vi "修改-探头报警值-网络版.vi"(7 "模式":enum16{"单项", "批量"}(ring), 8 "error in (no error)":errorcluster caption="错误输入（无错误）", 11 "探头属性 i":T1) -> (0 "error out":errorcluster caption="错误输出", 1 "取消?":bool=TRUE, 3 "探头属性 o":T1)   [LabVIEW 2017]
panel:
  in  "静音延迟":u16=5 min=5
  in  "报警方式选择":enum16{"常报警", "自动静音", "手动静音"}(ring)
  in  "累积限值":dbl=0.5 min=0.0 max=65536.0 format="%#_6f"
  in  "硬件报警等级":enum16{"一级限值", "二级限值"}(ring)
  in  "限值2":sgl=0.5 min=0 max=6553.6 format="%#.2f"
  in  "单位2":enum8{"uSv/h", "mSv/h"}(ring)
  in  "取消按钮":bool
  in  "确定按钮":bool
  in  "限值1":sgl=0.5 min=0 max=6553.6 format="%#.2f"
  in  "单位1":enum8{"uSv/h", "mSv/h"}(ring)
  # "剂量率限值"
  # "一级报警限值"
  # "二级报警限值"
  # "探头报警限值"
  # "报警与静音"
  # "静音延迟(秒)"
  # "自然累积剂量限值"
  # "累积报警限值"
  # "mSv"
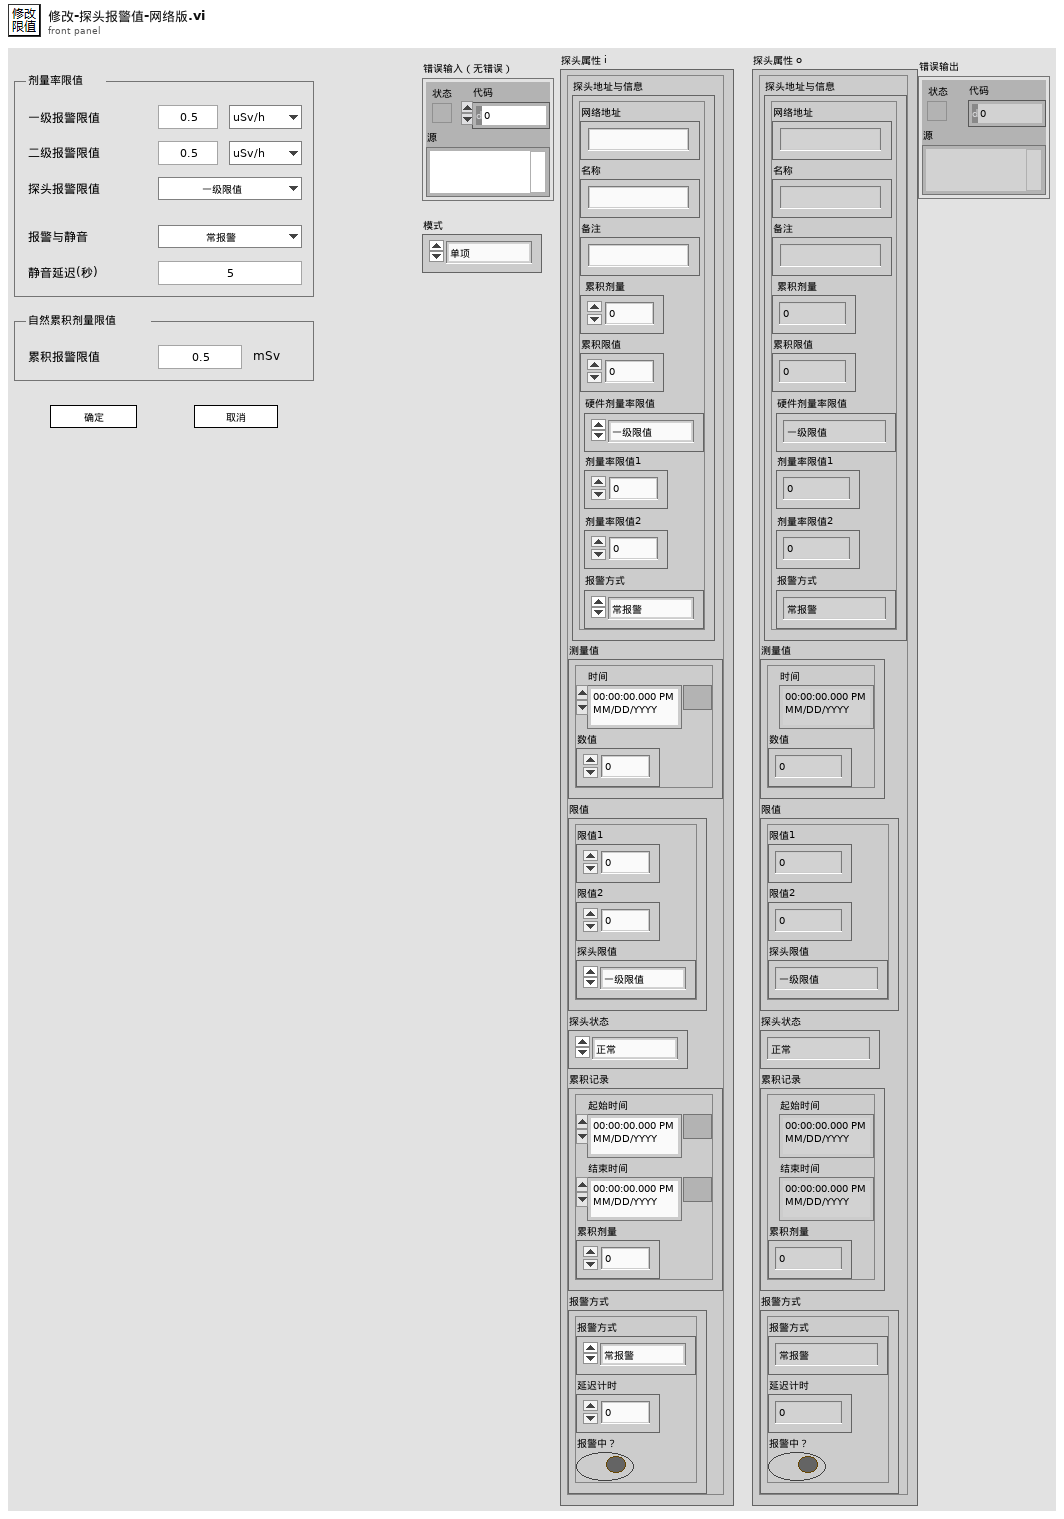
[diagram p1: front panel]
types:
  T1 = typedef "探头属性.ctl" = cluster{"探头地址与信息":T2, "测量值":T5, "限值":T6, "探头状态":T7, "累积记录":T8, "报警方式":T9}
  T2 = typedef "探测器信息.ctl" = cluster{"网络地址":string, "名称":string, "备注":string, "累积剂量":dbl, "累积限值":dbl, "硬件剂量率限值":T3, "剂量率限值1":dbl, "剂量率限值2":dbl, "报警方式":T4}
  T3 = typedef "探头剂量率限值选择.ctl" = enum16{"一级限值", "二级限值"}
  T4 = typedef "报警方式选择.ctl" = enum16{"常报警", "自动静音", "手动静音"}
  T5 = typedef "测量值.ctl" = cluster{"时间":timestamp, "数值":dbl}
  T6 = typedef "剂量率限值.ctl" = cluster{"限值1":dbl, "限值2":dbl, "探头限值":T3}
  T7 = typedef "探头状态.ctl" = enum16{"正常", "离线", "禁用", "一级报警", "二级报警", "累积报警"}
  T8 = typedef "单条累积记录.ctl" = cluster{"起始时间":timestamp, "结束时间":timestamp, "累积剂量":dbl}
  T9 = typedef "报警方式.ctl" = cluster{"报警方式":T4, "延迟计时":u16, "报警中？":bool}
  T10 = enum32{"Invalid", "Standard", "Closed", "Hidden", "Minimized", "Maximized"}
  T11 = enum8{"Enabled", "Disabled", "Disabled and Grayed Out"}
  T12 = typedef "簇-输入.ctl" = cluster{"配置文件动作":T13, "数据输入":variant}
  T13 = typedef "枚举-配置文件动作.ctl" = enum16{"初始化加载配置", "读取配置", "写入-屏幕键盘", "写入-静音延迟", "写入-主要探头类型", "写入-串口配置", "写入-累积定时", "写入-导出定时", "保存配置到文件"}
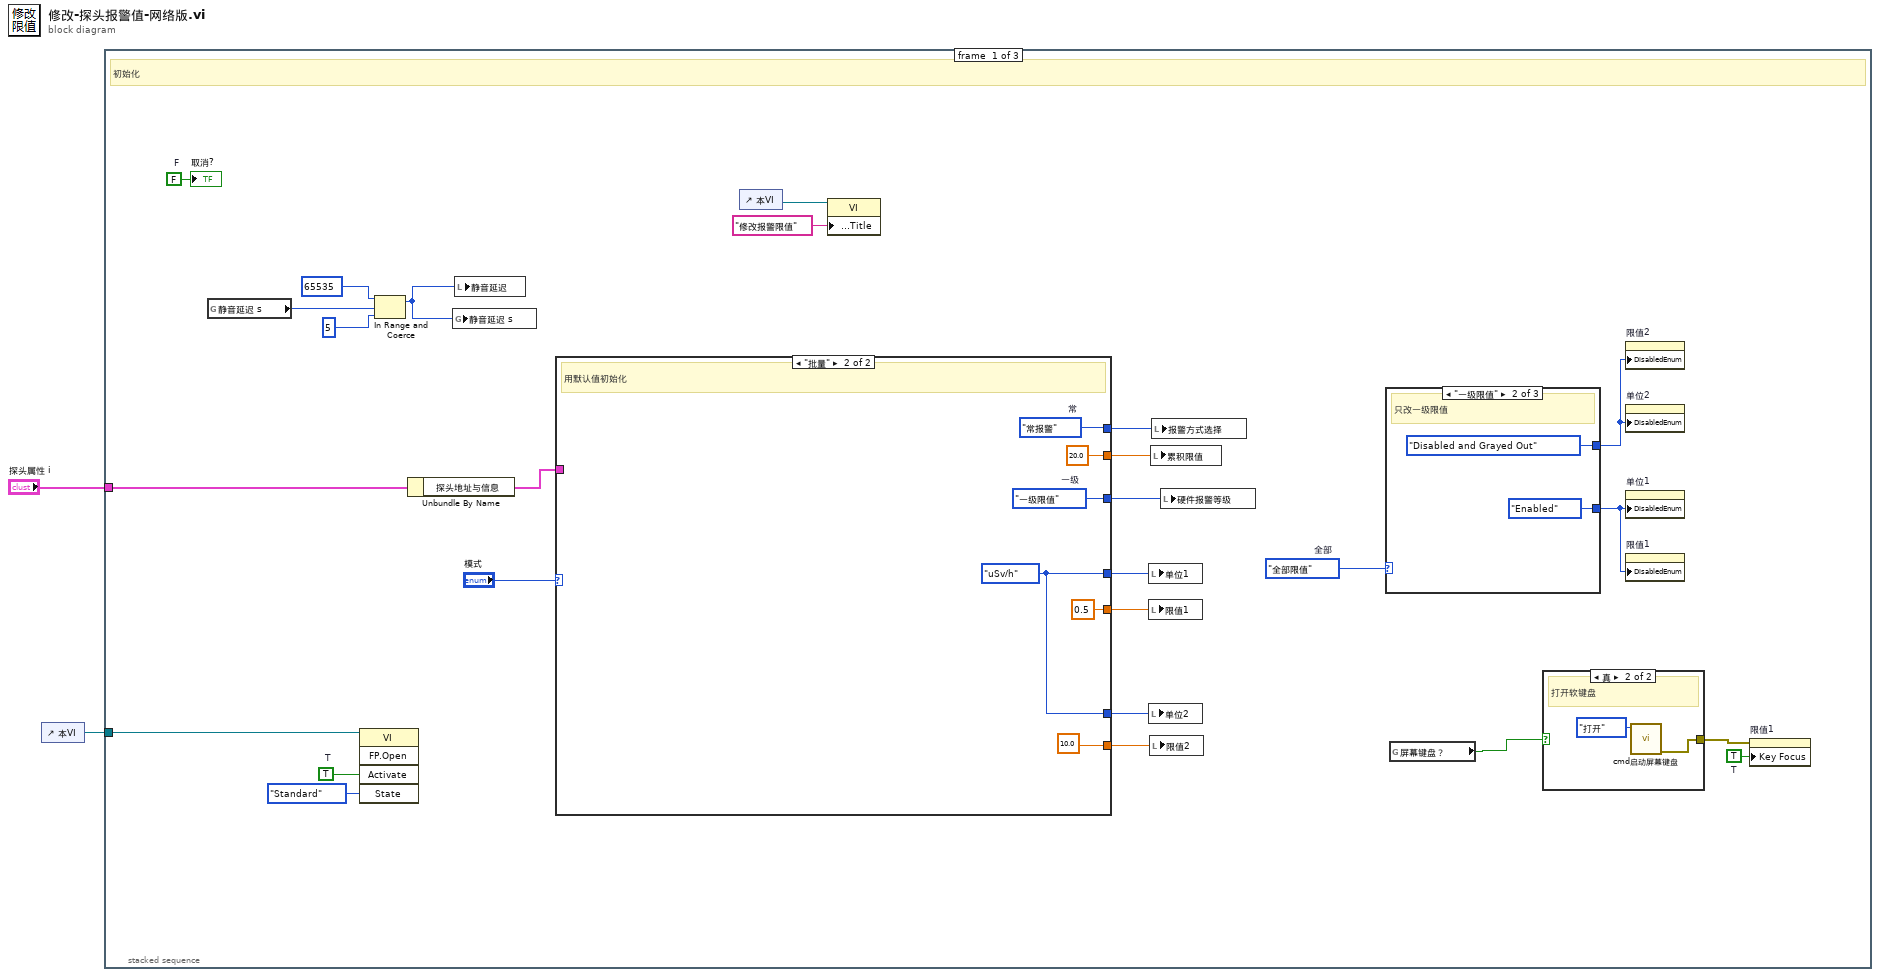
[diagram p0: block diagram]
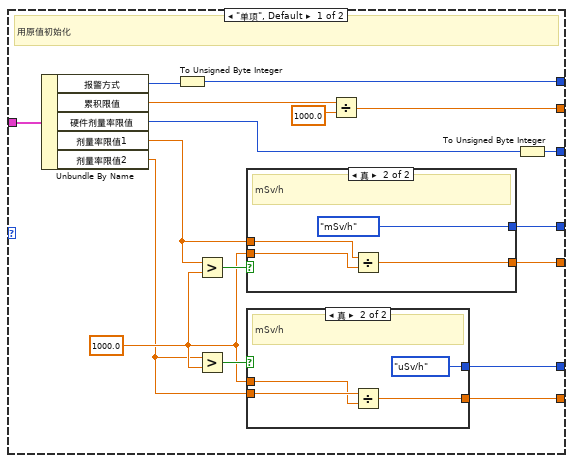
[diagram p2: hidden frame]
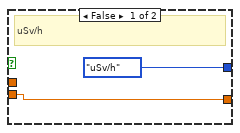
[diagram p3: hidden frame]
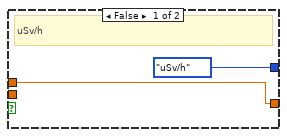
[diagram p4: hidden frame]
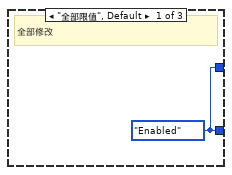
[diagram p6: hidden frame]
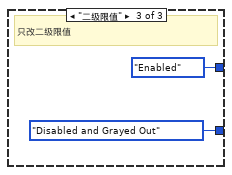
[diagram p7: hidden frame]
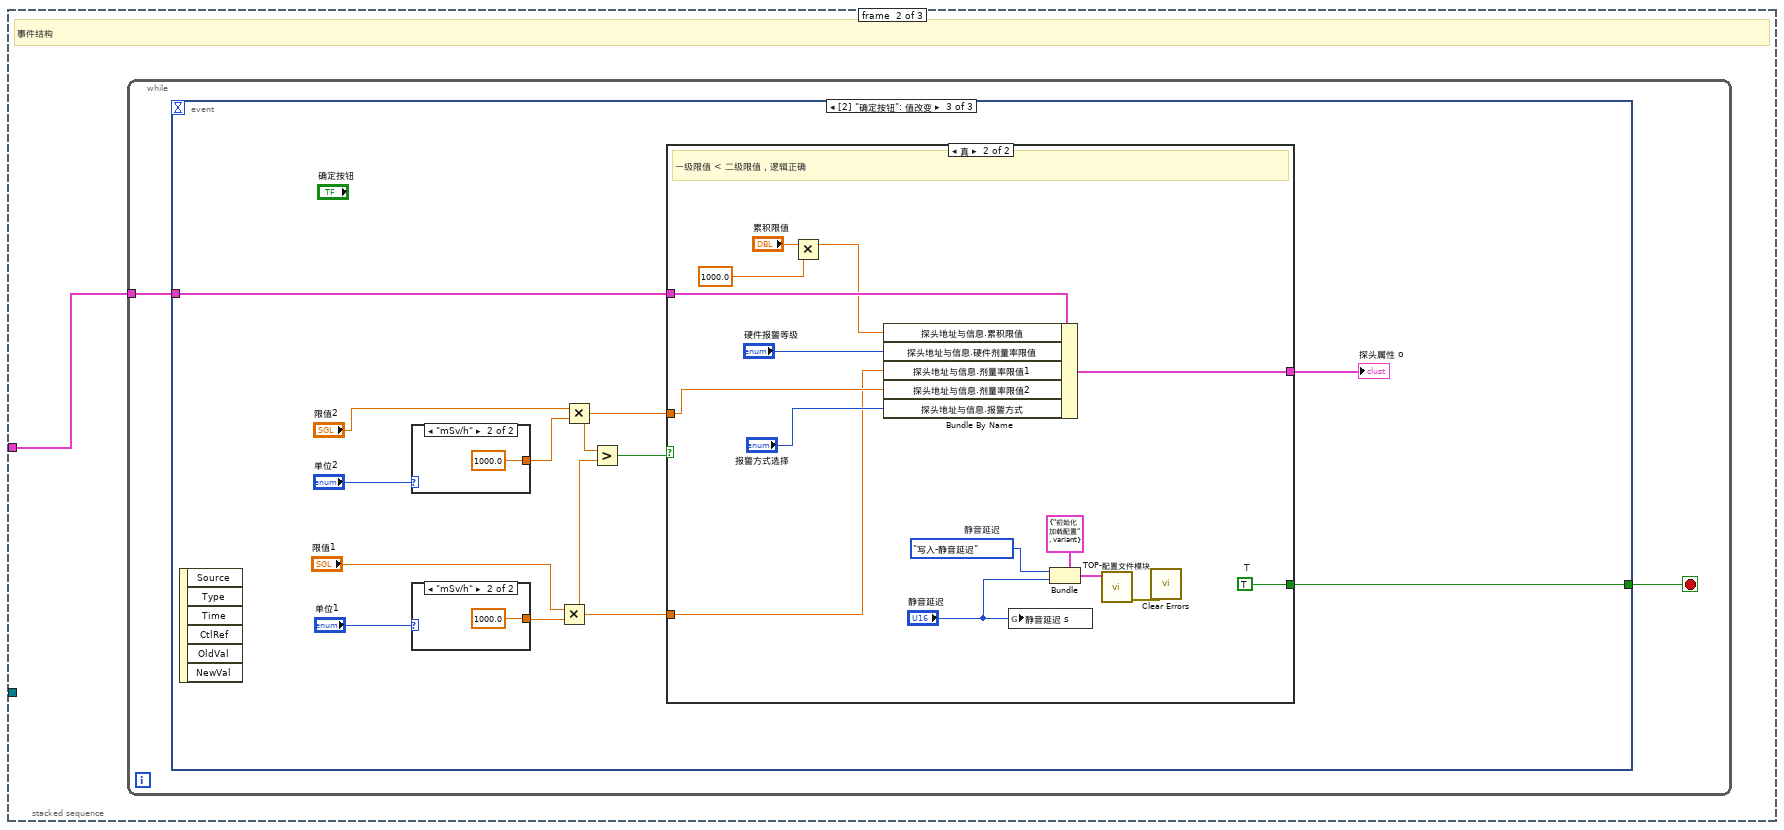
[diagram p8: hidden frame]
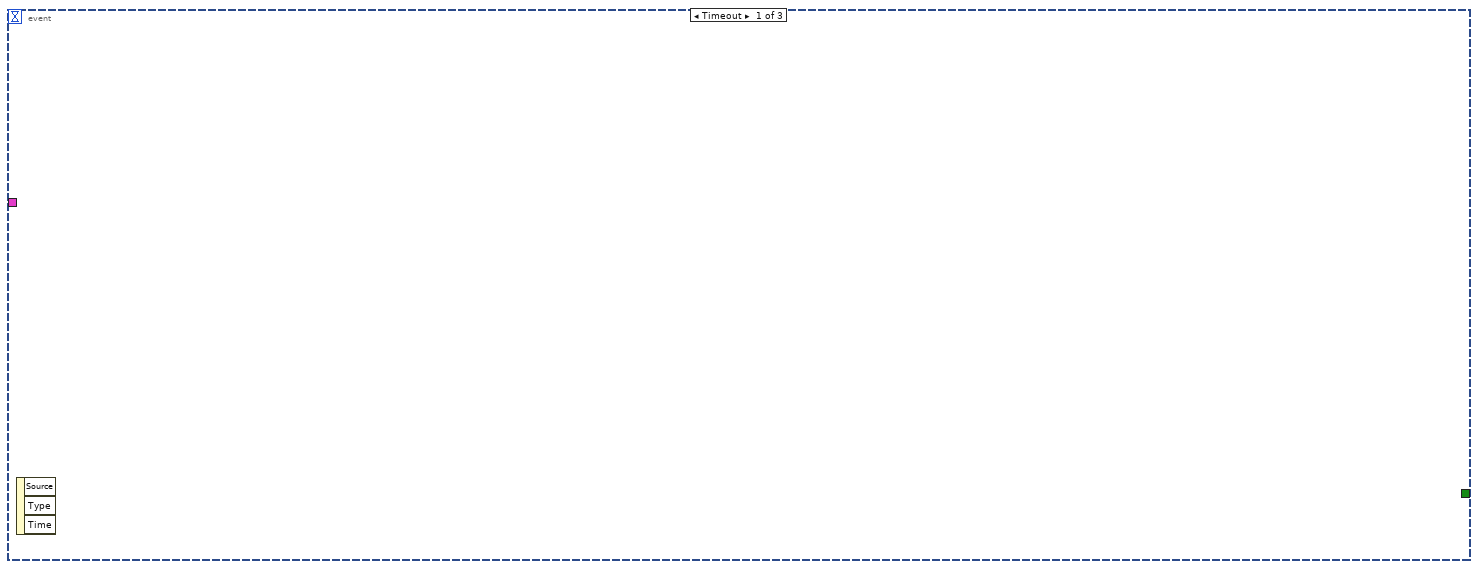
[diagram p9: hidden frame]
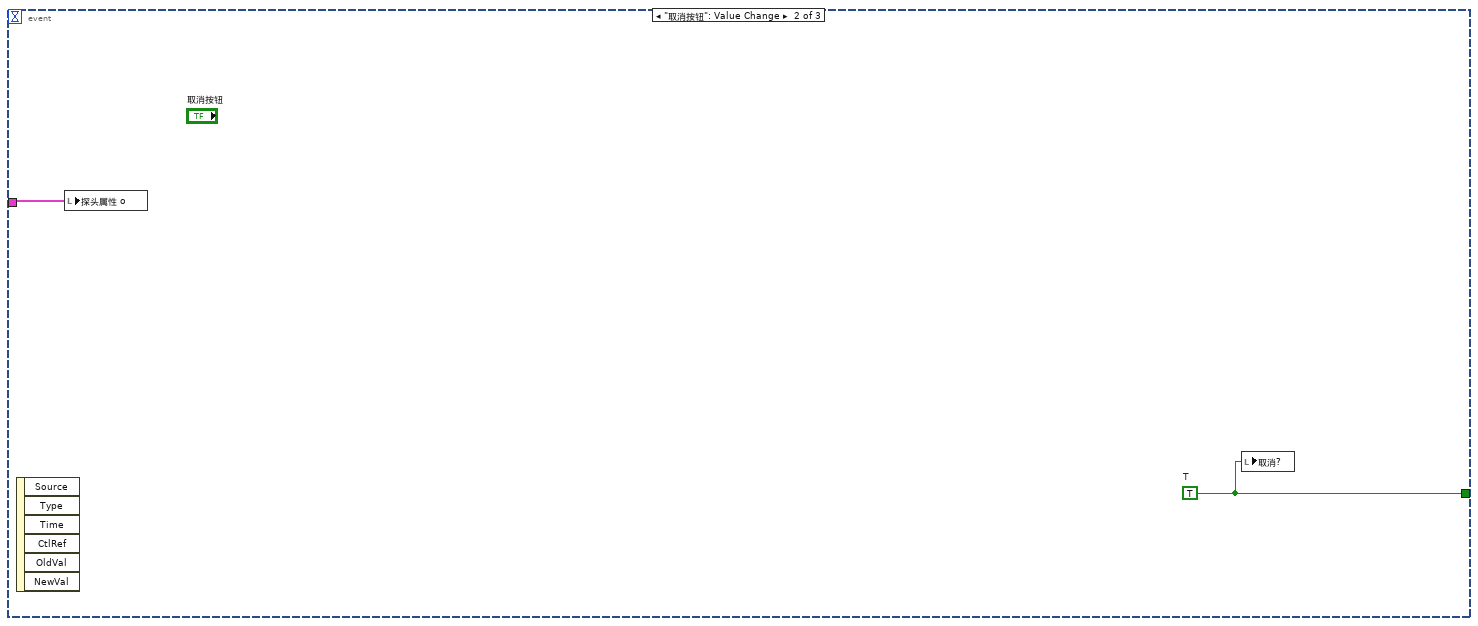
[diagram p10: hidden frame]
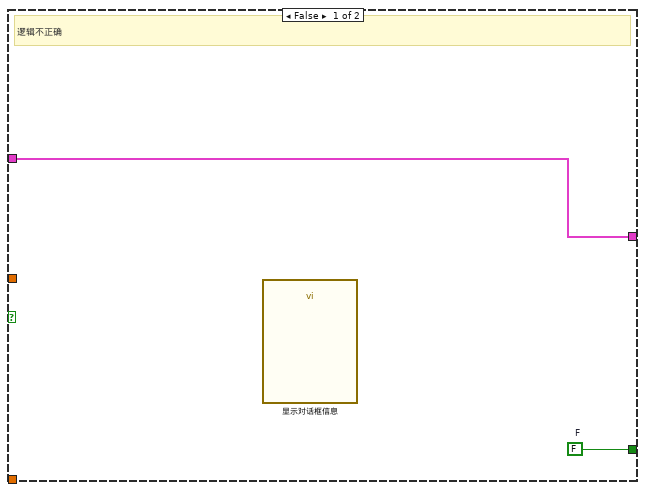
[diagram p11: hidden frame]
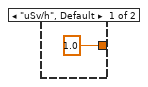
[diagram p12: hidden frame]
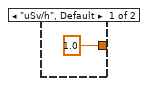
[diagram p13: hidden frame]
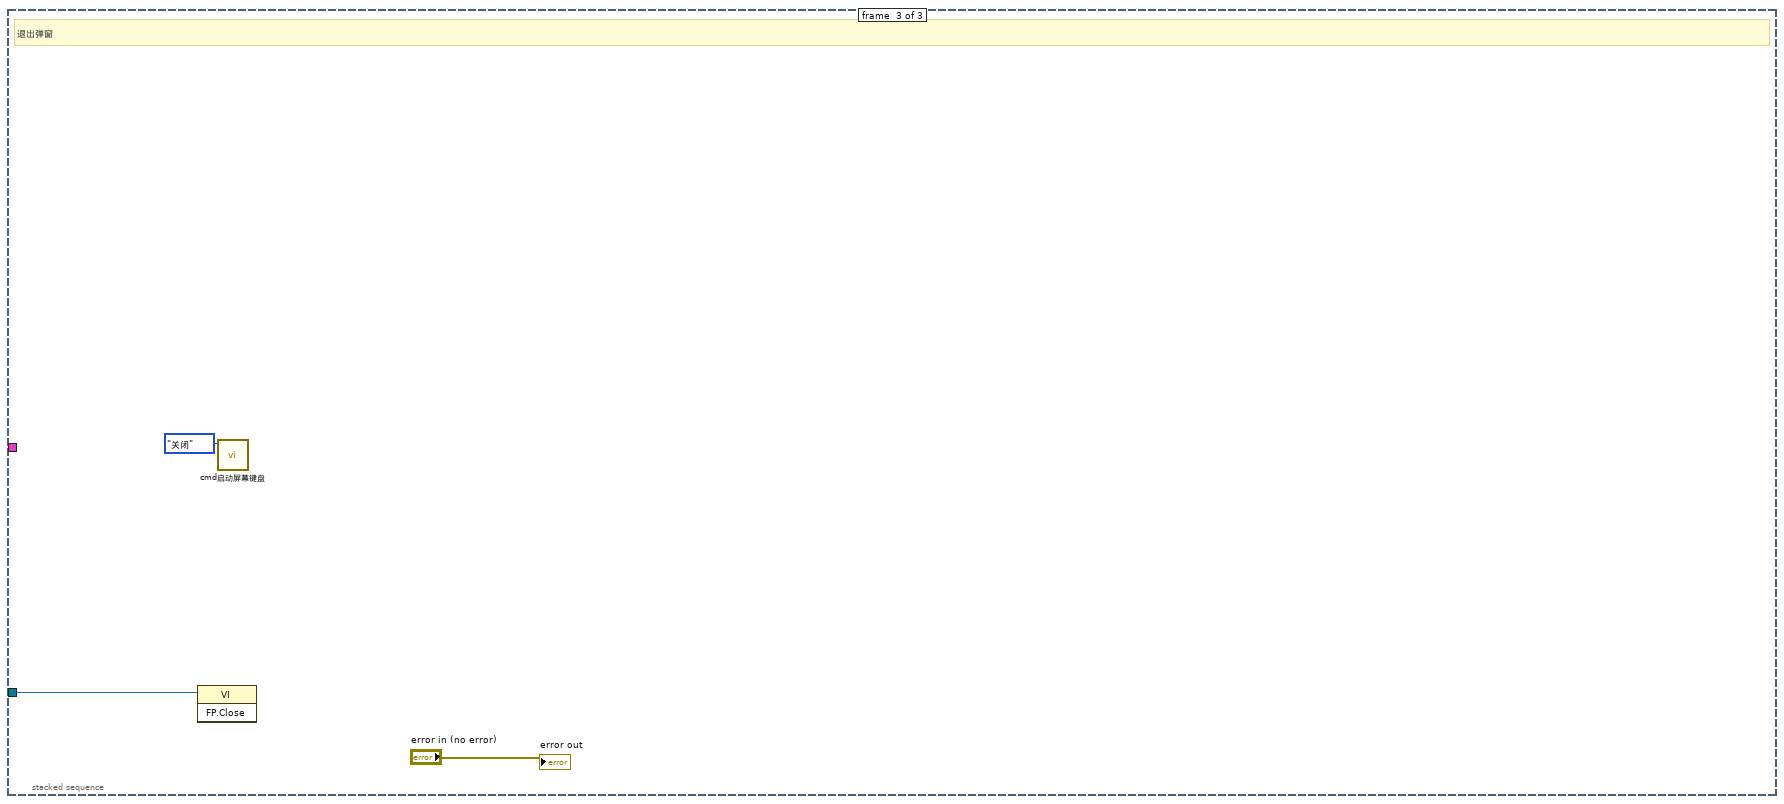
[diagram p14: hidden frame]
diagram:
  n1 = control-ref of="本VI"() -> (w2:refnum<vi>)
  n2 = stacked-sequence {
    tunnel: w2 -> [w26 _ w111]
    tunnel: "探头属性 i" -> [w15 w71 _]
    frame #0 {
      w3 = FALSE  # F
      w13 = TRUE  # T
      w19 = enum16{"全部限值", "一级限值", "二级限值"}."全部限值"  # 全部
      w28 = TRUE  # T
      # "初始化"
      n3 = global read "全局变量-35点监测.vi" "静音延迟 s"() -> (w7:u16)
      n4 = invoke class="VI" method="FP.Open"(reference=w26, "Activate"=w28, "State"=T10."Standard" ("状态")) -> ()  [unwired: 2 in, 5 out]
      n5 = In Range and Coerce(upper limit=u16 65535 ("y"), x=w7, lower limit=u16 5 ("y")) -> (coerced(x)=w4:u16)  [unwired: 1 out]
      n6 = Unbundle By Name(w15) -> ("探头地址与信息"=w11:T2)
      n7 = global write "全局变量-35点监测.vi" "静音延迟 s"(w4) -> ()
      n8 = local write "静音延迟"(w4) -> ()
      n9 = case shown="\"批量\"" "模式" {
        tunnel: [w45 0.5 ("剂量率限值1")] -> w25
        tunnel: [w44 w59] -> w24
        tunnel: [w43 w59] -> w23
        tunnel: [w42 10.0 ("剂量率限值1")] -> w22
        tunnel: [w31 w61] -> w8
        tunnel: [w30 20.0 ("累积限值")] -> w14
        tunnel: w11 -> [w34 _]
        tunnel: [w32 w63] -> w10
        frame "单项", Default {
          w38 = 1000.0 ("y")
          # "用原值初始化"
          n10 = Unbundle By Name(w34) -> ("报警方式"=w33:T4, "累积限值"=w35:dbl, "硬件剂量率限值"=w41:T3, "剂量率限值1"=w37:dbl, "剂量率限值2"=w36:dbl)
          n11 = To Unsigned Byte Integer(number=w33) -> (unsigned 8bit integer=w32:u8)
          n12 = Greater?(x=w37, y=w38) -> (0:w39:bool)
          n13 = Greater?(x=w36, y=w38) -> (0:w40:bool)
          n14 = case shown="真" w39 {
            tunnel: w37 -> [w52 w56]
            tunnel: w38 -> [_ w55]
            tunnel: [w52 w54] -> w45
            tunnel: [enum8{"uSv/h", "mSv/h"}."uSv/h" ("单位1") enum8{"uSv/h", "mSv/h"}."mSv/h" ("单位1")] -> w44
            frame False {
              # "uSv/h"
            }
            frame True {
              # "mSv/h"
              n15 = Divide(x=w56, y=w55) -> (x/y=w54:dbl)
            }
          }
          n16 = case shown="真" w40 {
            tunnel: w36 -> [w46 w50]
            tunnel: w38 -> [_ w49]
            tunnel: [enum8{"uSv/h", "mSv/h"}."uSv/h" ("单位1") enum8{"uSv/h", "mSv/h"}."uSv/h" ("单位1")] -> w43
            tunnel: [w46 w48] -> w42
            frame False {
              # "uSv/h"
            }
            frame True {
              # "mSv/h"
              n17 = Divide(x=w50, y=w49) -> (x/y=w48:dbl)
            }
          }
          n18 = Divide(x=w35, y=1000.0 ("x")) -> (x/y=w30:dbl)
          n19 = To Unsigned Byte Integer(number=w41) -> (unsigned 8bit integer=w31:u8)
        }
        frame "批量" {
          w59 = enum8{"uSv/h", "mSv/h"}."uSv/h" ("单位1")
          w61 = enum16{"一级限值", "二级限值"}."一级限值"  # 一级
          w63 = enum16{"常报警", "自动静音", "手动静音"}."常报警"  # 常
          # "用默认值初始化"
        }
      }
      n20 = control-ref of="本VI"() -> (w17:refnum<vi>)
      n21 = property class="VI"(reference=w17, "Front Panel.Title"="修改报警限值" ("前面板窗口:标题")) -> ()  [unwired: 1 in, 2 out]
      n22 = local write "单位1"(w24) -> ()
      n23 = local write "限值1"(w25) -> ()
      n24 = local write "单位2"(w23) -> ()
      n25 = local write "限值2"(w22) -> ()
      n26 = local write "累积限值"(w14) -> ()
      n27 = local write "报警方式选择"(w10) -> ()
      n28 = local write "硬件报警等级"(w8) -> ()
      n29 = case shown="\"一级限值\"" w19 {
        tunnel: [w66 T11."Enabled" ("禁用") T11."Disabled and Grayed Out" ("禁用")] -> w21
        tunnel: [w66 T11."Disabled and Grayed Out" ("禁用") T11."Enabled" ("禁用")] -> w20
        frame "全部限值", Default {
          w66 = T11."Enabled" ("禁用")
          # "全部修改"
        }
        frame "一级限值" {
          # "只改一级限值"
        }
        frame "二级限值" {
          # "只改二级限值"
        }
      }
      n30 = global read "全局变量-35点监测.vi" "屏幕键盘？"() -> (w18:bool)
      n31 = case shown="真" w18 {
        tunnel: [_ w64] -> w12
        frame False {
        }
        frame True {
          # "打开软键盘"
          n32 = call "cmd启动屏幕键盘.vi"("软键盘开关"=enum16{"关闭", "打开"}."打开") -> ("error out"=w64:errorcluster)  [unwired: 9 in, 1 out]
        }
      }
      n33 = property on="限值2" class="DigNum (严格)"("DisabledEnum"=w20) -> ()  [unwired: 2 in, 2 out]
      n34 = property on="单位2" class="Enum (严格)"("DisabledEnum"=w20) -> ()  [unwired: 2 in, 2 out]
      n35 = property on="单位1" class="Enum (严格)"("DisabledEnum"=w21) -> ()  [unwired: 2 in, 2 out]
      n36 = property on="限值1" class="DigNum (严格)"("DisabledEnum"=w21) -> ()  [unwired: 2 in, 2 out]
      n37 = property on="限值1" class="DigNum (严格)"(error in=w12, "Key Focus"=w13) -> ()  [unwired: 1 in, 2 out]
      "取消?" <- w3
    }
    frame #1 {
      # "事件结构"
      n38 = while {
        tunnel: w71 -> [w72]
        stop <- w73 stop-if-true
        n39 = event shown="[2] \"确定按钮\": 值改变" {
          selector: _ -> [_ _ _]
          dyn-events: _ -> [_ _ _]
          timeout: _ -> [_ _ _]
          tunnel: [_ w74 w83] -> w73
          tunnel: w72 -> [_ w75 w77]
          event Timeout {
            n40 = event-data() -> ()  [unwired: 1 in, 3 out]
          }
          event "取消按钮": Value Change {
            w74 = TRUE  # T
            n41 = event-data() -> ()  [unwired: 1 in, 6 out]
            n42 = local write "探头属性 o"(w75) -> ()
            n43 = local write "取消?"(w74) -> ()
          }
          event "确定按钮": Value Change {
            n44 = event-data() -> ()  [unwired: 1 in, 6 out]
            n45 = case shown="\"mSv/h\"" "单位2" {
              tunnel: [sgl 1.0 ("探头报警值") sgl 1000.0 ("探头报警值")] -> w81
              frame "uSv/h", Default {
              }
              frame "mSv/h" {
              }
            }
            n46 = case shown="\"mSv/h\"" "单位1" {
              tunnel: [sgl 1.0 ("探头报警值") sgl 1000.0 ("探头报警值")] -> w82
              frame "uSv/h", Default {
              }
              frame "mSv/h" {
              }
            }
            n47 = Multiply(x="限值1", y=w82) -> (x*y=w78:sgl)
            n48 = Multiply(x="限值2", y=w81) -> (x*y=w79:sgl)
            n49 = Greater?(x=w79, y=w78) -> (0:w80:bool)
            n50 = case shown="真" w80 {
              tunnel: w78 -> [_ w98]
              tunnel: w79 -> [_ w99]
              tunnel: [w89 w104] -> w83
              tunnel: w77 -> [w88 w103]
              tunnel: [w88 w97] -> w76
              frame False {
                w89 = FALSE  # F
                # "逻辑不正确"
                n51 = call "显示对话框信息"() -> ()  [unwired: 10 in, 2 out]
              }
              frame True {
                w93 = 枚举-配置文件动作."写入-静音延迟"  # 静音延迟
                w104 = TRUE  # T
                # "一级限值 < 二级限值，逻辑正确"
                n52 = Multiply(x="累积限值", y=1000.0) -> (x*y=w96:dbl)
                n53 = Bundle By Name(cluster=w103, "探头地址与信息.累积限值"=w96, "探头地址与信息.硬件剂量率限值"="硬件报警等级", "探头地址与信息.剂量率限值1"=w98, "探头地址与信息.剂量率限值2"=w99, "探头地址与信息.报警方式"="报警方式选择") -> (w97:T1)
                n54 = global write "全局变量-35点监测.vi" "静音延迟 s"("静音延迟") -> ()
                n55 = Bundle(cluster=T12 {"配置文件动作"=enum."初始化加载配置", "数据输入"=variant} ("输入"), "配置文件动作"=w93, "数据输入"="静音延迟") -> (w94:T12)
                n56 = call "TOP-配置文件模块.vi"("输入"=w94) -> ("error out"=w90:errorcluster)  [unwired: 9 in, 1 out]
                n57 = call <vilib>:"Clear Errors.vi"("error in (no error)"=w90) -> ()  [unwired: 5 in, 2 out]
              }
            }
            "探头属性 o" <- w76
          }
        }
      }
    }
    frame #2 {
      # "退出弹窗"
      n58 = invoke class="VI" method="FP.Close"(reference=w111) -> ()  [unwired: 2 in, 3 out]
      n59 = call "cmd启动屏幕键盘.vi"("软键盘开关"=enum16{"关闭", "打开"}."关闭") -> ()  [unwired: 9 in, 2 out]
      "error out" <- "error in (no error)"
    }
  }
